vi "Python Node Test.vi"() -> ()   [LabVIEW 2025]
doc: "This example demonstrates how to call a Python function and pass doubles as arguments. It uses a python function to compute the sum of two doubles."
uses:
  Program Files/National Instruments/LabVIEW 2025/examples/Connectivity/Python/support/PythonVersionsEnum.ctl
  <vilib>/Python/Open Anaconda Python Session.vi
panel:
  out "Waveform Chart":dbl(graph)
  in  "stop":bool
  out "Numeric":i32=2
  out "Results":T1={"reading"=20736.0, "polarity"="Positive", "enable"=FALSE} {"reading" format="%#_6p"}
  in  "cal_file":string="C:\\Engineering\\Hexium\\Rydberg\\Source Code\\Instrument Drivers\\Spectrometer Prototype\\Cal_SPA120.json"
  in  "Port":string="COM6"
  in  "Parameters":T2={"channel"=1, "range_index"=2, "bias"=0.0, "sample_rate"=10, "samples"=5}
  out "error out":errorcluster
  in  "error in":errorcluster
  in  "Python version":T3=enum."3.10"
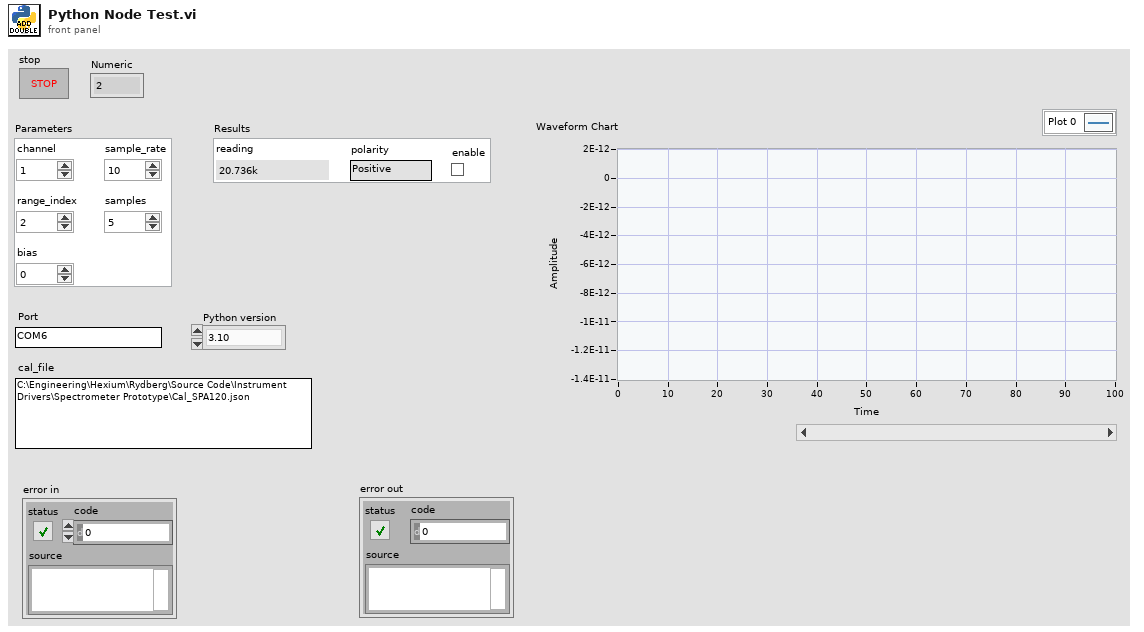
[diagram p1: front panel]
types:
  T1 = cluster{"reading":dbl, "polarity":string, "enable":bool}
  T2 = cluster{"channel":i32, "range_index":i32, "bias":dbl, "sample_rate":i32, "samples":i32}
  T3 = typedef "PythonVersionsEnum.ctl" = enum16{"3.6", "3.7", "3.8", "3.9", "3.10"}
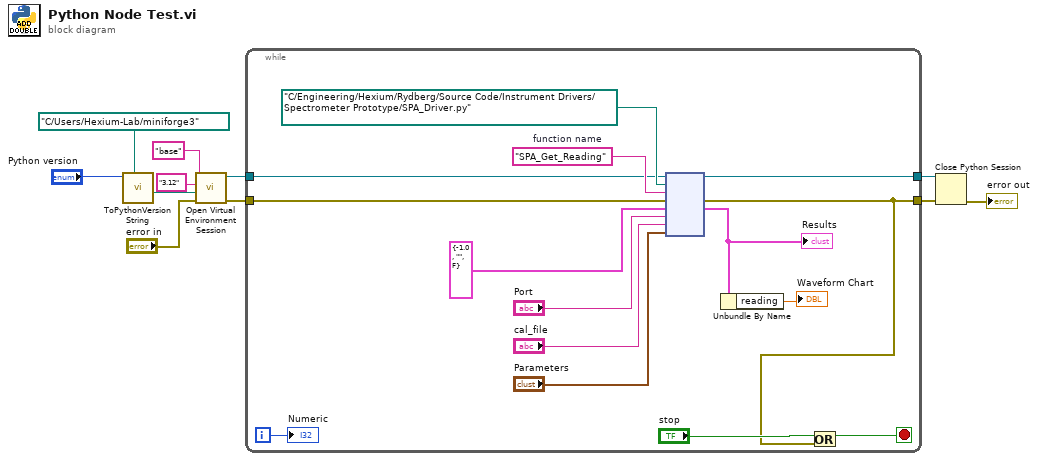
[diagram p0: block diagram]
diagram:
  n1 = call "ToPythonVersionString.vi"("python version"="Python version") -> ()  [unwired: 10 in, 1 out]
  n2 = call-poly <vilib>:"Open Virtual Environment Session.vi"("error in (no error)"="error in", "Anaconda path"=path "C:/Users/Hexium-Lab/miniforge3" ("Python path"), "Python version"="3.12", "Env name"="base") -> ("error out"=w8:errorcluster, "session out"=w9:refnum<k35>)  [unwired: 6 in]
  n3 = while {
    tunnel: w9 -> [w18]
    tunnel: w8 -> [w17]
    tunnel: [w16] -> w5
    tunnel: [w13] -> w4
    i -> [w19]
    stop <- w14 stop-if-true
    w25 = "SPA_Get_Reading"  # function name
    n4 = node(w18, path "C:/Engineering/Hexium/Rydberg/Source Code/Instrument Drivers/Spectrometer Prototype/SPA_Driver.py" ("module path"), w25, w17, T1 {"reading"=-1.0, "polarity"="", "enable"=FALSE} ("Results"), "Port", "cal_file", "Parameters") -> (w16:refnum<k35>, w13:errorcluster, w11:T1)  [unwired: 3 in, 2 out]
    "Results" <- w11
    n5 = Unbundle By Name(w11) -> ("reading"=→"Waveform Chart":dbl)
    n6 = Or(x="stop", y=w13) -> (x .or. y?=w14:bool)
    "Numeric" <- w19
  }
  n7 = Close Python Session(session in=w5, error in=w4) -> (11:→"error out":errorcluster)
